vi "Custom_Append VI Icon to Report (path).vi"(0 "report in":refnum<class "NI_report.lvclass">, 2 "image format (jpeg)":enum32{"PNG", "JPEG", "GIF"}(ring)=enum."JPEG", 5 "VI":path, 7 "alignment (default)":T1, 9 "caption or alternative string":string, 11 "error in (no error)":errorcluster, 12 "MS Office parameters":T2) -> (4 "report out":refnum<class "NI_report.lvclass">, 6 "VI path out":path, 8 "start out (Word)":i32, 10 "end out (Word)":i32, 15 "error out":errorcluster)   [LabVIEW 2019]
doc: "Appends the icon of the VI you specify in <B>VI</B> to a report. Wire data to the <B>VI</B> input to determine the polymorphic instance to use or manually select the instance."
uses:
  <vilib>/Utility/NIReport.llb/NI_report.lvclass
  <vilib>/Utility/NIReport.llb/HTML Report Image Alignment.ctl
  <vilib>/Utility/NIReport.llb/NI_ReportGenerationCore.lvlib
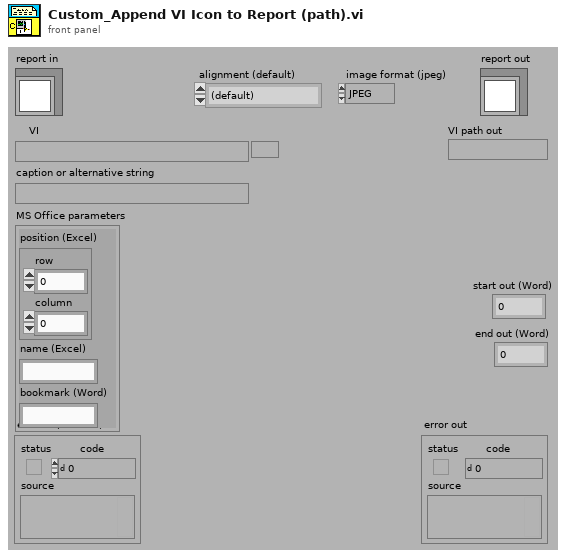
[diagram p1: front panel]
types:
  T1 = typedef "NI_ReportGenerationCore.lvlib/HTML Report Image Alignment.ctl" = enum16{"(default)", "LEFT", "RIGHT", "TOP", "TEXTTOP", "MIDDLE", "ABSMIDDLE", "BASELINE", "BOTTOM", "ABSBOTTOM"}
  T2 = cluster{"position (Excel)":cluster{"row":i32, "column":i32}, "name (Excel)":string, "bookmark (Word)":string}
  T3 = enum32{"invalid app kind", "Development System", "Run Time System", "Student Edition", "Embedded LabVIEW", "Evaluation", "Custom"}
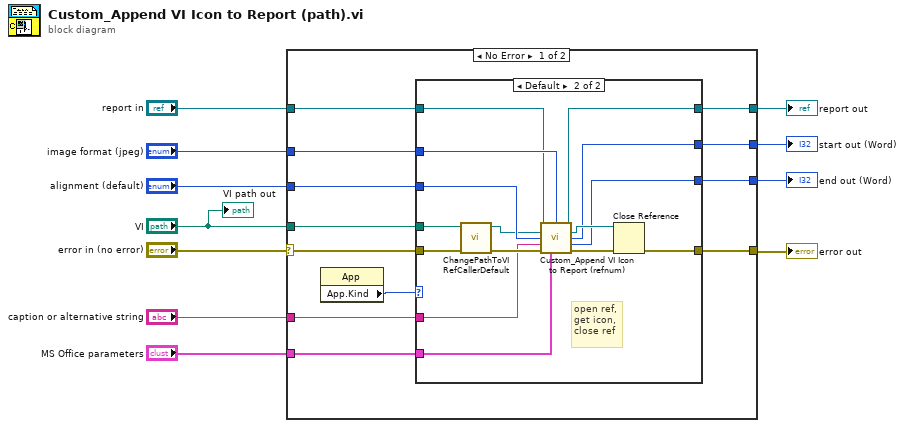
[diagram p0: block diagram]
diagram:
  n1 = case shown="No Error" "error in (no error)" {
    selector: "error in (no error)" -> [w21 w42]
    tunnel: [w17 w42] -> w10
    tunnel: [w22 w41] -> w8
    tunnel: "report in" -> [w23 w41]
    tunnel: "VI" -> [w14 _]
    tunnel: "image format (jpeg)" -> [w18 _]
    tunnel: "MS Office parameters" -> [w20 _]
    tunnel: "alignment (default)" -> [w19 _]
    tunnel: [w16 _] -> w3
    tunnel: [w15 _] -> w2
    tunnel: "caption or alternative string" -> [w13 _]
    frame No Error {
      n2 = property class="App"() -> ("App.Kind"=w12:T3)  [unwired: 2 in, 2 out]
      n3 = case shown="Default" w12 {
        tunnel: w23 -> [w25 w26]
        tunnel: [w25 w29] -> w22
        tunnel: w21 -> [w24 w40]
        tunnel: w20 -> [_ w38]
        tunnel: w19 -> [_ w37]
        tunnel: w18 -> [_ w36]
        tunnel: [w24 w34] -> w17
        tunnel: [_ w32] -> w16
        tunnel: [_ w28] -> w15
        tunnel: w14 -> [_ w30]
        tunnel: w13 -> [_ w27]
        frame "Run Time System" {
          # "Do not try to append\nif running in an\nexecutable"
        }
        frame Default {
          # "open ref,\nget icon,\nclose ref"
          n4 = call <vilib>:"ChangePathToVIRefCallerDefault.vi"("error in (no error)"=w40, "VI path"=w30) -> ("error out"=w39:errorcluster, "VI reference"=w31:refnum<vi>)  [unwired: 4 in]
          n5 = call "Custom_Append VI Icon to Report (refnum).vi"("report in"=w26, "image format (jpeg)"=w36, "VI"=w31, "alignment (default)"=w37, "caption or alternative string"=w27, "error in (no error)"=w39, "MS Office parameters"=w38) -> ("report out"=w29:refnum<class "NI_report.lvclass">, "VI out"=w33:refnum<vi>, "start out (Word)"=w32:i32, "end out (Word)"=w28:i32, "error out"=w35:errorcluster)  [unwired: 4 in]
          n6 = Close Reference(reference=w33, error in (no error)=w35) -> (error out=w34:errorcluster)
        }
      }
    }
    frame Error {
    }
  }
  "error out" <- w10
  "report out" <- w8
  "start out (Word)" <- w3
  "end out (Word)" <- w2
  "VI path out" <- "VI"
